vi "InitialiseDevice.vi"(8 "error In":errorcluster, 9 "PicoMotor IP In":string) -> (0 "error out":errorcluster, 1 "Device Address Out":i32, 2 "DeviceKey Out":string, 3 "CmdLib Out":refnum<k24>)   [LabVIEW 2020]
uses:
  C:/GEECS/Developers Version/source/Device Drivers/Picomotor8742dotNet/NewFocus/CmdLib.dll
  NewFocus/CmdLib.dll
panel:
  out "index of element":i32
  out "DeviceKey List Out":string[](array[string])
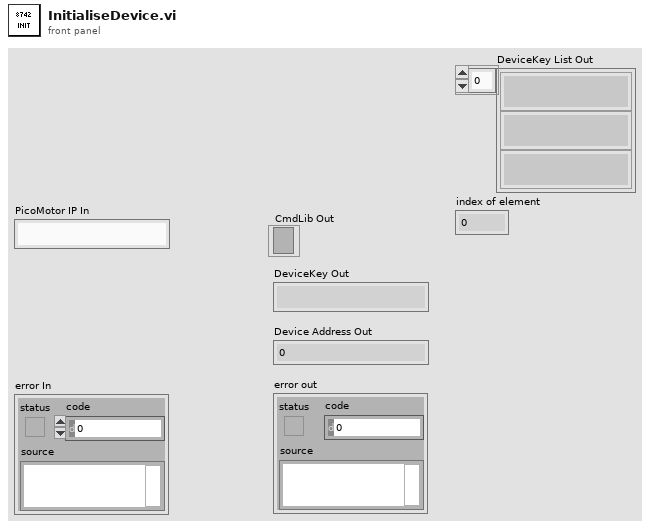
[diagram p1: front panel]
types:
  T1 = cluster{"DeviceKey":string, "Device Address":i32, "Controller Name":string}[]
  T2 = cluster{"DeviceKey":string, "Device Address":i32, "Controller Name":string}
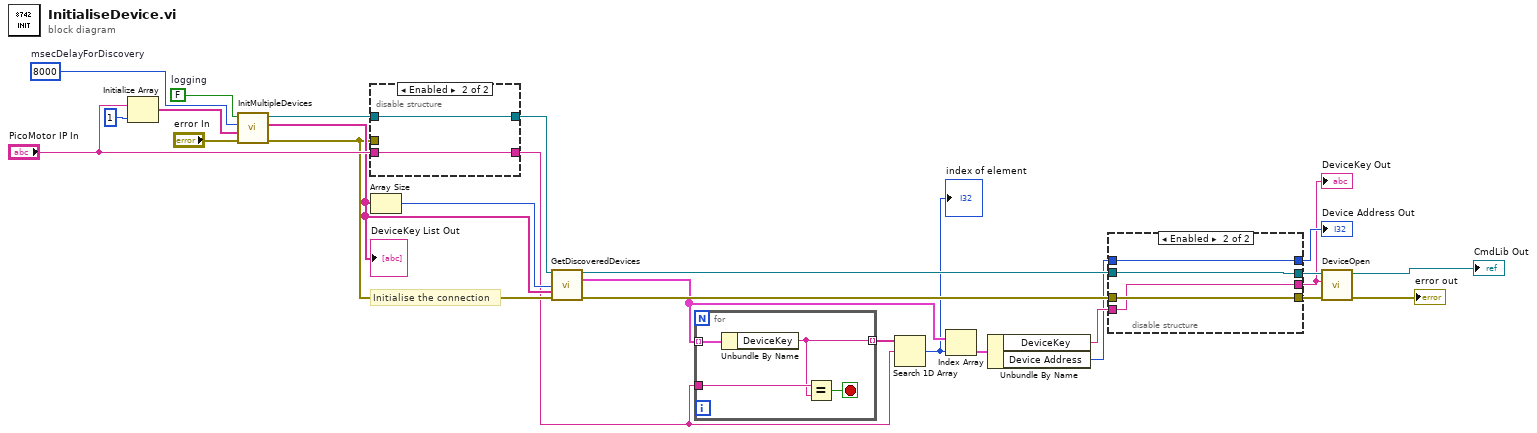
[diagram p0: block diagram]
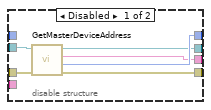
[diagram p2: hidden frame]
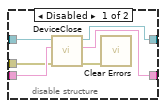
[diagram p3: hidden frame]
diagram:
  w21 = FALSE  # logging
  w26 = 8000  # msecDelayForDiscovery
  # "Initialise the connection"
  n1 = Initialize Array("PicoMotor IP In", 1 ("dimension size")) -> (w25:string[])
  n2 = call "InitMultipleDevices.vi"("error in (no error)"="error In", "deviceKeys"=w25, "msecDelayForDiscovery"=w26, "logging"=w21) -> ("error out"=w9:errorcluster, "DeviceKey List Out"=w11:string[], "CmdLib Out"=w20:refnum<k24>)  [unwired: 1 in]
  "DeviceKey List Out" <- w11
  n3 = disable-structure shown="Enabled" {
    disable-tunnel: w20 -> [w32 w34]
    disable-tunnel: [w31 w34] -> w13
    disable-tunnel: "PicoMotor IP In" -> [w30 w33]
    disable-tunnel: [w29 w33] -> w6
    disable-tunnel: w9 -> [w27 _]
    frame Disabled {
      n4 = call "DeviceClose.vi"("error in (no error)"=w27, "DeviceKey In"=w30, "CmdLib In"=w32) -> ("error out"=w28:errorcluster, "DeviceKey Out"=w29:string, "CmdLib Out"=w31:refnum<k24>)  [unwired: 2 in]
      n5 = call <vilib>:"Clear Errors.vi"("error in (no error)"=w28) -> ()  [unwired: 5 in, 2 out]
    }
    frame Enabled {
    }
  }
  n6 = Array Size(array=w11) -> (size(s)=w10:i32)
  n7 = call "GetDiscoveredDevices.vi"("CmdLib In"=w13, "Master Count"=w10, "DeviceKey List"=w11, "error in"=w9) -> ("CmdLib Out"=w12:refnum<k24>, "Device Array"=w5:T1, "error out"=w8:errorcluster)  [unwired: 9 in]
  n8 = for {
    tunnel: w5 -> [w38] mode=indexing
    tunnel: w6 -> [w37]
    tunnel: [w35] -> w7 mode=indexing
    stop <- w36 stop-if-true
    n9 = Unbundle By Name(w38) -> ("DeviceKey"=w35:string)
    n10 = Equal?(x=w37, y=w35) -> (x = y?=w36:bool)
  }
  n11 = Search 1D Array(1D array=w7, element=w6) -> (index of element=w4:i32)  [unwired: 1 in]
  "index of element" <- w4
  n12 = Index Array(array=w5, index=w4) -> (element=w3:T2)
  n13 = Unbundle By Name(w3) -> ("DeviceKey"=w2:string, "Device Address"=w1:i32)
  n14 = disable-structure shown="Enabled" {
    disable-tunnel: [w44 w45] -> w23
    disable-tunnel: [w43 w48] -> w18
    disable-tunnel: [w42 w46] -> w17
    disable-tunnel: [w41 w47] -> w16
    disable-tunnel: w12 -> [w40 w48]
    disable-tunnel: w8 -> [w39 w47]
    disable-tunnel: w2 -> [_ w46]
    disable-tunnel: w1 -> [_ w45]
    frame Disabled {
      n15 = call "GetMasterDeviceAddress.vi"("error in (no error)"=w39, "CmdLib In"=w40) -> ("error out"=w41:errorcluster, "Device Address"=w44:i32, "DeviceKey Out"=w42:string, "CmdLib Out"=w43:refnum<k24>)  [unwired: 2 in]
    }
    frame Enabled {
    }
  }
  "Device Address Out" <- w23
  "DeviceKey Out" <- w17
  n16 = call "DeviceOpen.vi"("error in (no error)"=w16, "DeviceKey In"=w17, "CmdLib In"=w18) -> ("error out"=→"error out":errorcluster, "CmdLib Out"=→"CmdLib Out":refnum<k24>)  [unwired: 2 in, 1 out]
